vi "Sequence.CompleteMain.vi"(7 "Code.Main":refnum<k24>, 8 "error in (no error)":errorcluster, 10 "Abort":T1, 11 "Refs":T2) -> (0 "error out":errorcluster)   [LabVIEW 2013, in "Simple Sequence Editor.lvlib"]
uses:
  Simple Sequence Editor.lvlib
  Types/Sequence.MainSeqRefs.ctl
  NationalInstruments.VeriStand.RealTimeSequenceDefinitionApi
  Types/ChannelProperties.ctl
  Constants.vi
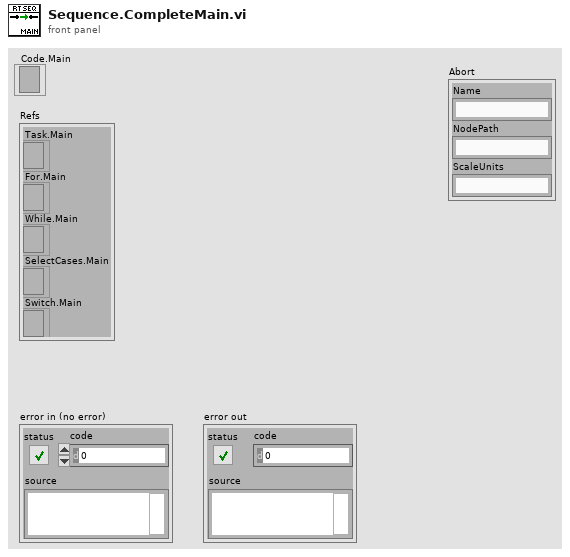
[diagram p1: front panel]
types:
  T1 = typedef "Simple Sequence Editor.lvlib/ChannelProperties.ctl" = cluster{"Name":string, "NodePath":string, "ScaleUnits":string}
  T2 = typedef "Simple Sequence Editor.lvlib/Sequence.MainSeqRefs.ctl" = cluster{"Task.Main":refnum<k24>, "For.Main":refnum<k24>, "While.Main":refnum<k24>, "SelectCases.Main":refnum<k24>, "Switch.Main":refnum<k24>}
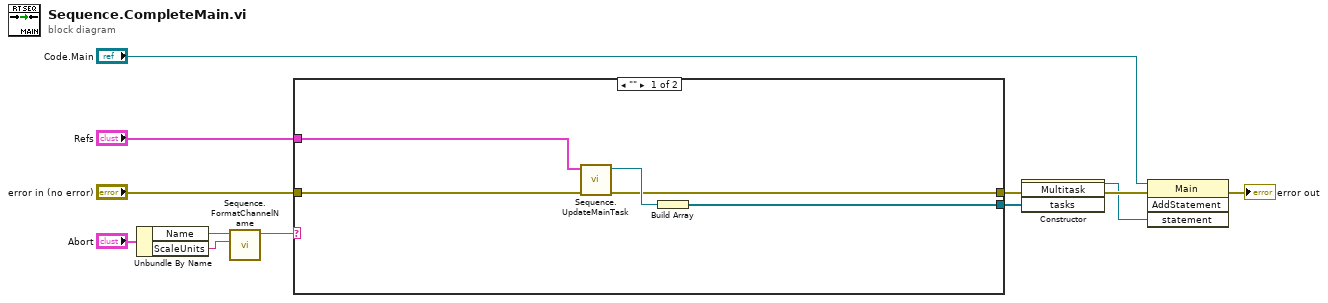
[diagram p0: block diagram]
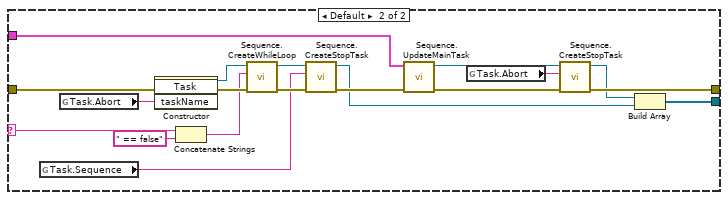
[diagram p2: hidden frame]
diagram:
  n1 = Unbundle By Name("Abort") -> ("Name"=w3:string, "ScaleUnits"=w4:string)
  n2 = call "Sequence.FormatChannelName.vi"("ScaleUnits"=w4, "Name"=w3) -> ("ChannelName"=w1:string)  [unwired: 9 in]
  n3 = case shown="\"\"" w1 {
    selector: w1 -> [_ w31]
    tunnel: "error in (no error)" -> [w15 w36]
    tunnel: [w13 w24] -> w8
    tunnel: [w17 w28] -> w7
    tunnel: "Refs" -> [w16 w18]
    frame "" {
      n4 = call "Sequence.UpdateMainTask.vi"("error in (no error)"=w15, "Refs"=w16) -> ("error out"=w13:errorcluster, "Task.Main Ref"=w14:refnum<k24>)  [unwired: 8 in]
      n5 = Build Array(w14) -> (w17:refnum<k24>[])
    }
    frame Default {
      n6 = global read "Constants.vi" "Task.Sequence"() -> (w21:string)
      n7 = global read "Constants.vi" "Task.Abort"() -> (w20:string)
      n8 = constructor class="Task"(error in=w36, "taskName"=w20) -> (reference out=w35:refnum<k24>, error out=w34:errorcluster)  [unwired: 2 in, 2 out]
      n9 = Concatenate Strings(w31, " == false" ("string")) -> (w29:string)
      n10 = call "Sequence.CreateWhileLoop.vi"("error in (no error)"=w34, "Expression"=w29, "Task Ref"=w35) -> ("error out"=w33:errorcluster, "Task Ref out"=w32:refnum<k24>)  [unwired: 7 in]
      n11 = call "Sequence.CreateStopTask.vi"("error in (no error)"=w33, "Task Name"=w21, "Task Ref"=w32) -> ("error out"=w27:errorcluster, ".NET Refnum out"=w22:refnum<k24>)  [unwired: 7 in]
      n12 = call "Sequence.UpdateMainTask.vi"("error in (no error)"=w27, "Refs"=w18) -> ("error out"=w25:errorcluster, "Task.Main Ref"=w26:refnum<k24>)  [unwired: 8 in]
      n13 = global read "Constants.vi" "Task.Abort"() -> (w19:string)
      n14 = call "Sequence.CreateStopTask.vi"("error in (no error)"=w25, "Task Name"=w19, "Task Ref"=w26) -> ("error out"=w24:errorcluster, ".NET Refnum out"=w23:refnum<k24>)  [unwired: 7 in]
      n15 = Build Array(w23, w22) -> (w28:refnum<k24>[])
    }
  }
  n16 = constructor class="Multitask"(error in=w8, "tasks"=w7) -> (reference out=w10:refnum<k24>, error out=w11:errorcluster)  [unwired: 2 in, 2 out]
  n17 = invoke class="Main" method="AddStatement"(reference="Code.Main", error in=w11, "statement"=w10) -> (error out=→"error out":errorcluster)  [unwired: 1 in, 3 out]
